vi "Check file size.vi"(8 "error in (no error)":errorcluster, 10 "min size (KB)":i64, 11 "DAQOrcaFlash in":refnum<class "DAQOrcaFlash.lvclass">) -> (0 "error out":errorcluster, 2 "too small?":bool, 3 "DAQOrcaFlash out":refnum<class "DAQOrcaFlash.lvclass">)   [LabVIEW 2012, in "DAQOrcaFlash.lvclass"]
uses:
  DAQOrcaFlash.lvclass
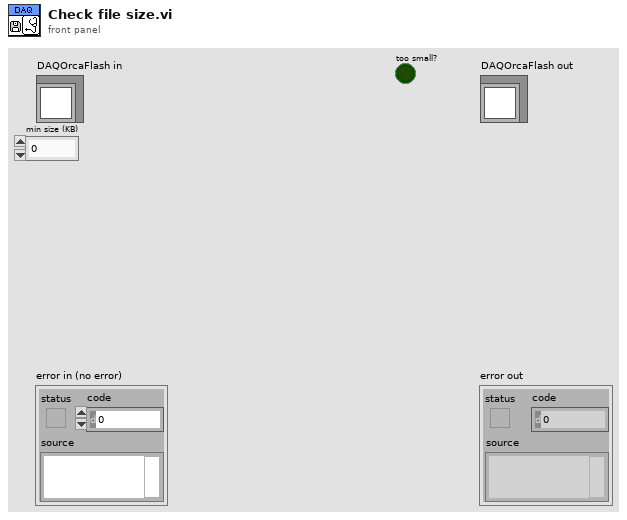
[diagram p1: front panel]
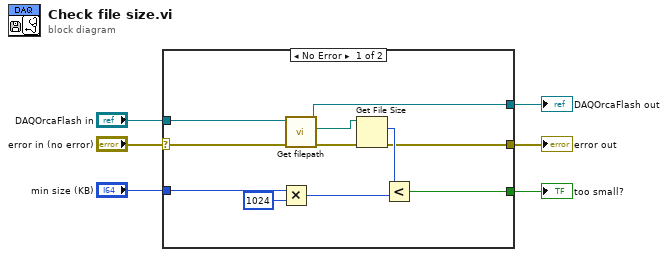
[diagram p0: block diagram]
diagram:
  n1 = case shown="No Error" "error in (no error)" {
    selector: "error in (no error)" -> [w11 w19]
    tunnel: [w12 w19] -> w5
    tunnel: [w9 w18] -> w3
    tunnel: "DAQOrcaFlash in" -> [w8 w18]
    tunnel: "min size (KB)" -> [w16 _]
    tunnel: [w13 _] -> w1
    frame No Error {
      n2 = Multiply(x=w16, y=i64 1024 ("size (in bytes)")) -> (x*y=w14:i64)
      n3 = call "Get filepath.vi"("error in (no error)"=w11, "DAQOrcaFlash in"=w8) -> ("error out"=w10:errorcluster, "full storage path"=w7:path, "DAQOrcaFlash out"=w9:refnum<class "DAQOrcaFlash.lvclass">)  [unwired: 7 in]
      n4 = Get File Size(file=w7, error in=w10) -> (size (in bytes)=w15:i64, 0:w12:errorcluster)  [unwired: 1 out]
      n5 = Less?(x=w15, y=w14) -> (x < y?=w13:bool)
    }
    frame Error {
    }
  }
  "error out" <- w5
  "DAQOrcaFlash out" <- w3
  "too small?" <- w1
